vi "Test_Dig_Wfm.vi"(8 "Plot Colors":u32[](array[numeric]), 9 "Threshold Value of a circuit":dbl=30.0, 11 "DataLog":path=path "/Macintosh HD/Users/hasan/My_MAC_Data/3_Dissemination/ICCAD 2016/Experimental_Data/Ckt 8 - Majority Muller C element/kd-0.0135/Majority Muller C_SSADataLog.xls") -> (2 "Close 2":bool)   [LabVIEW 2014]
uses:
  <vilib>/Utility/file.llb/Read From Spreadsheet File (DBL).vi
  <vilib>/Utility/file.llb/Read From Spreadsheet File (string).vi
  <vilib>/Waveform/DTblOps.llb/DTbl Boolean Array to Digital.vi
panel:
  out "size(s)":i32
  out "x/y":dbl
  out "Clr":u32[](array[numeric])
  out "x-scale-multiplier":dbl=10.0
  out "Digital Waveform Graph 2":digitaldata[](graph)
  out "Digital":path
  out "Time":dbl[](array[numeric])
  out "Thres vals":dbl[](array[numeric])
  out "Int Time":i32[](array[numeric])
  out "Idx":i32[](array[numeric])
  out "Q":i32
  out "floor(x/y)":dbl
  out "Plot Names":string[](array[string])=["A", "B", "C", "P0", "P1", "P10", "P11", "P12", "P13", "P2", "P3", "P4", "P5", "P6", "P7", "P8", "P9", "S1", "S2", "S3", "S4", "X", "Y", "Z"]
  out "Mixed Signal Graph":T1(graph)
  out "x > y?":bool[][](array[boolean])
  out "Sp Data":dbl[][](array[numeric]) format="%0.3f"
  in  "Cancel Button":bool
  in  "Close":bool
  in  "Reset":bool
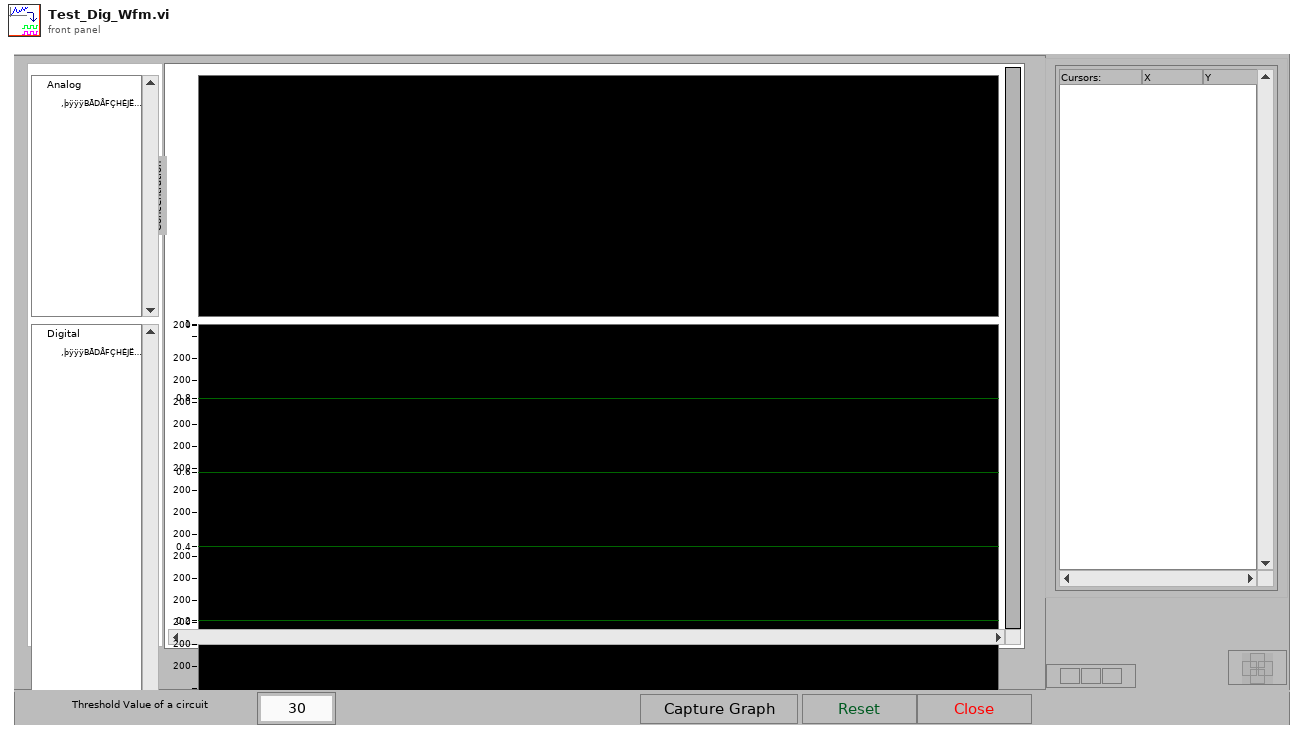
[diagram p1: front panel]
types:
  T1 = cluster{cluster{"Time":i32[], dbl[]}[], digitaldata[]}
  T2 = cluster{cluster{"Int Time":i32[], dbl[]}[], digitaldata[]}
  T3 = cluster{"Color":u32, "PointStyle":u8, "LineStyle":u8, "Interp":u8, "LineWidth":u8, "BarPlotStyle":u8, "FillTo":i16, "XScaleIdx":u32, "YScaleIdx":u32, "Anti-Aliased":bool, "LabelFormat":u8, "TransitionType":u8, "TransitionLocation":u8, "DigitalLineStyle":u8}
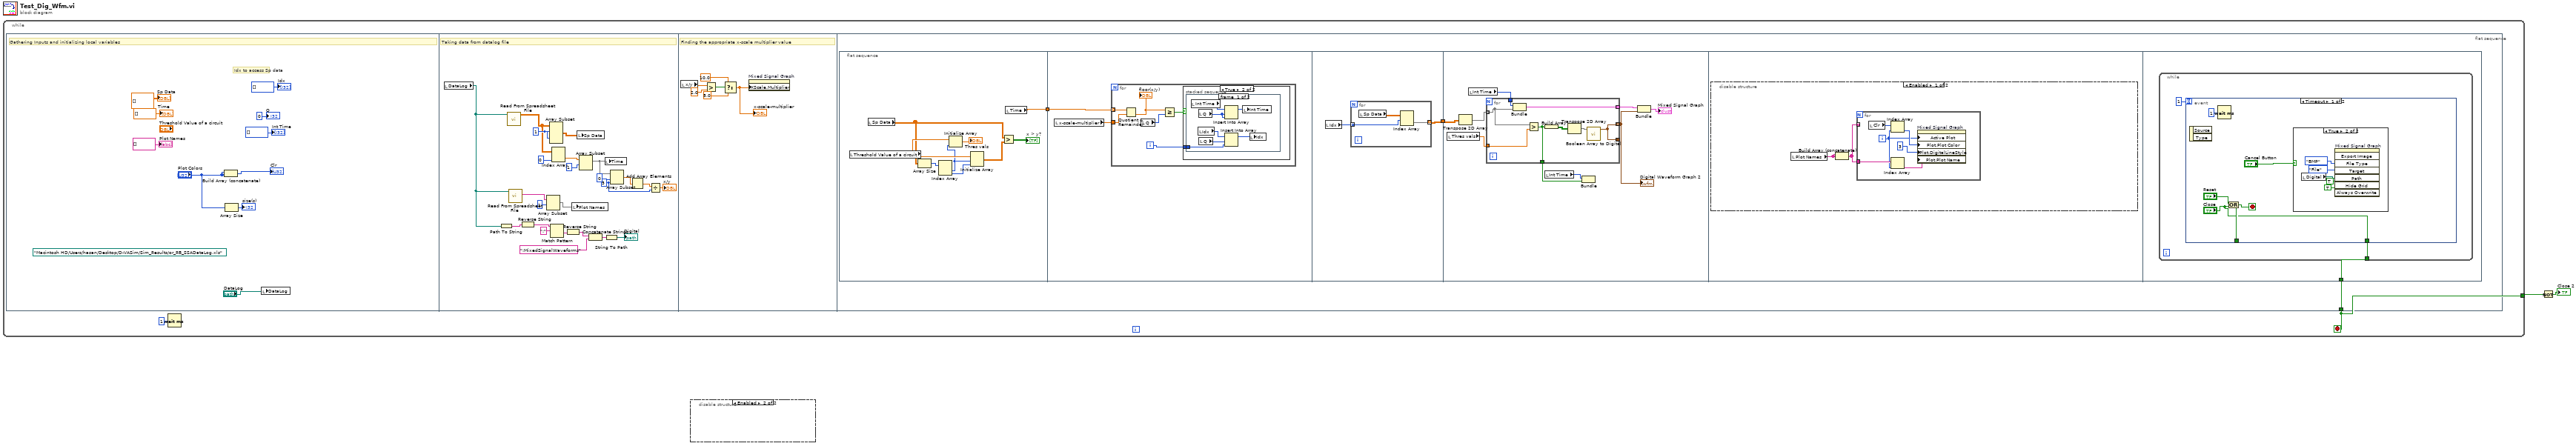
[diagram p0: block diagram]
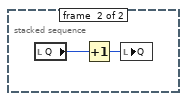
[diagram p3: hidden frame]
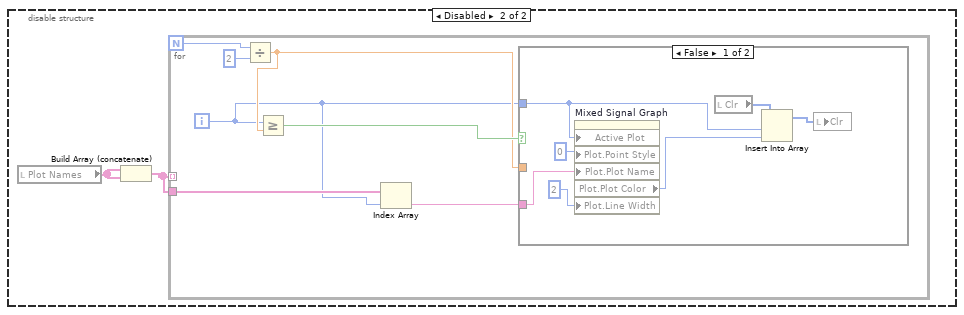
[diagram p4: hidden frame]
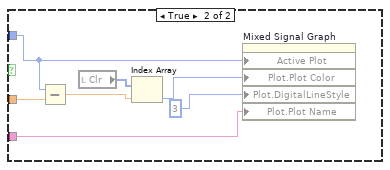
[diagram p5: hidden frame]
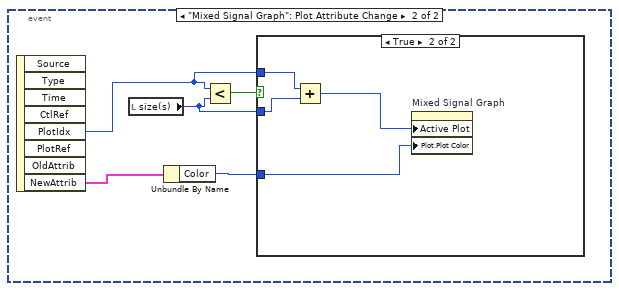
[diagram p7: hidden frame]
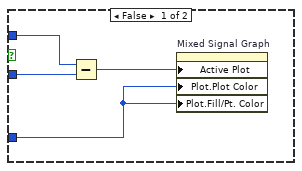
[diagram p8: hidden frame]
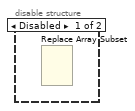
[diagram p9: hidden frame]
diagram:
  n1 = while {
    tunnel: [w3] -> w2
    stop <- w3 stop-if-true
    n2 = flat-sequence {
      tunnel: [w45] -> w3
      frame #0 {
        (unwired) path "/Macintosh HD/Users/hasan/Desktop/D-VASim/Sim_Results/or_RB_SSADataLog.xls" ("DataLog")
        # "Idx to access Sp data"
        # "Gathering Inputs and initializing local variables"
        n3 = Build Array (concatenate)("Plot Colors", "Plot Colors") -> (→"Clr":u32[])
        n4 = Array Size(array="Plot Colors") -> (size(s)=→"size(s)":i32)
        n5 = local write "DataLog"("DataLog") -> ()
        "Sp Data" <- dbl[][] [] ("Sp Data")
        "Plot Names" <- string[] [] ("Plot Names")
        "Time" <- dbl[] [] ("Time")
        "Idx" <- i32[] []
        "Q" <- 0
        "Int Time" <- i32[] []
      }
      frame #1 {
        w16 = 5 ("length")
        w38 = 1 ("index")
        # "Taking data from datalog file"
        n6 = local read "DataLog"() -> (w21:path)
        n7 = Path To String(path=w21) -> (string=w23:string)
        n8 = call-poly <vilib>:"Read From Spreadsheet File.vi"("file path (dialog if empty)"=w21) -> ("all rows"=w36:dbl[][])  [unwired: 6 in, 4 out]
        n9 = call-poly <vilib>:"Read From Spreadsheet File.vi"("file path (dialog if empty)"=w21) -> ("first row"=w32:string[])  [unwired: 6 in, 4 out]
        n10 = Reverse String(1:w23) -> (0:w24:string)
        n11 = Array Subset(array=w32, index=1) -> (w31:string[])  [unwired: 1 in]
        n12 = Array Subset(array=w36, index (row)=w38, index (col)=w38) -> (w37:dbl[][])  [unwired: 2 in]
        n13 = Match Pattern(string=w24, regular expression=":") -> (after substring=w26:string)  [unwired: 1 in, 3 out]
        n14 = Index Array(array=w36, index (col)=0 ("index")) -> (element=w34:dbl[])  [unwired: 1 in]
        n15 = Reverse String(1:w26) -> (0:w27:string)
        n16 = local write "Plot Names"(w31) -> ()
        n17 = local write "Sp Data"(w37) -> ()
        n18 = Array Subset(array=w34, index=1) -> (w20:dbl[])  [unwired: 1 in]
        n19 = Concatenate Strings(w27, ":MixedSignalWaveforms" ("regular expression")) -> (w29:string)
        n20 = local write "Time"(w20) -> ()
        n21 = String To Path(string=w29) -> (path=→"Digital":path)
        n22 = Array Subset(array=w20, index=0, length=w16) -> (w18:dbl[])
        n23 = Add Array Elements(numeric array=w18) -> (sum=w17:dbl)
        n24 = Divide(x=w17, y=w16) -> (x/y=→"x/y":dbl)
      }
      frame #2 {
        # "Finding the appropriate x-scale multiplier value"
        n25 = local read "x/y"() -> (w44:dbl)
        n26 = Greater?(x=w44, y=2.0) -> (0:w42:bool)
        n27 = Select(t=10.0, s=w42, f=5.0) -> (s? t:f=w39:dbl)
        "x-scale-multiplier" <- w39
        n28 = property on="Mixed Signal Graph" class="MixedGraph (strict)"("XScale.Multiplier"=w39) -> ()  [unwired: 2 in, 2 out]
      }
      frame #3 {
        n29 = flat-sequence {
          tunnel: [w56] -> w46
          tunnel: w46 -> [w58]
          tunnel: [w75] -> w47
          tunnel: w47 -> [w85]
          tunnel: [w128] -> w45
          frame #0 {
            n30 = local read "Threshold Value of a circuit"() -> (w55:dbl)
            n31 = local read "Sp Data"() -> (w54:dbl[][])
            n32 = Array Size(array=w54) -> (size(s)=w49:i32[])
            n33 = Index Array(array=w49) -> (element #1=w52:i32, element #2=w48:i32)  [unwired: 2 in]
            n34 = Initialize Array(w55, w52) -> (→"Thres vals":dbl[])
            n35 = Initialize Array(w55, w52, w48) -> (w50:dbl[][])
            n36 = Greater?(x=w54, y=w50) -> (0:→"x > y?":bool[][])
            n37 = local read "Time"() -> (w56:dbl[])
          }
          frame #1 {
            n38 = local read "x-scale-multiplier"() -> (w57:dbl)
            n39 = for {
              tunnel: w58 -> [w64] mode=indexing
              tunnel: w57 -> [w61]
              i -> [w62]
              n40 = Quotient & Remainder(x=w64, y=w61) -> (floor(x/y)=w60:dbl)  [unwired: 1 out]
              "floor(x/y)" <- w60
              n41 = local read "Q"() -> (w59:i32)
              n42 = Greater Or Equal?(x=w60, y=w59) -> (x >= y?=w63:bool)
              n43 = case shown="True" w63 {
                tunnel: w62 -> [_ w65]
                frame False {
                }
                frame True {
                  n44 = stacked-sequence {
                    tunnel: w65 -> [w66 _]
                    frame #0 {
                      n45 = local read "Int Time"() -> (w72:i32[])
                      n46 = local read "Idx"() -> (w67:i32[])
                      n47 = local read "Q"() -> (w70:i32)
                      n48 = local read "Q"() -> (w69:i32)
                      n49 = Insert Into Array(array=w72, index=w70, new element=w70) -> (w71:i32[])
                      n50 = Insert Into Array(array=w67, index=w69, new element=w66) -> (w68:i32[])
                      n51 = local write "Int Time"(w71) -> ()
                      n52 = local write "Idx"(w68) -> ()
                    }
                    frame #1 {
                      n53 = local read "Q"() -> (w74:i32)
                      n54 = Increment(x=w74) -> (x+1=w73:i32)
                      n55 = local write "Q"(w73) -> ()
                    }
                  }
                }
              }
            }
          }
          frame #2 {
            n56 = local read "Idx"() -> (w76:i32[])
            n57 = for {
              tunnel: w76 -> [w78] mode=indexing
              tunnel: [w77] -> w75 mode=indexing
              n58 = local read "Sp Data"() -> (w79:dbl[][])
              n59 = Index Array(array=w79, index (row)=w78) -> (element=w77:dbl[])  [unwired: 1 in]
            }
          }
          frame #3 {
            n60 = local read "Thres vals"() -> (w88:dbl[])
            n61 = Transpose 2D Array(2D array=w85) -> (transposed array=w87:dbl[][])
            n62 = local read "Int Time"() -> (w84:i32[])
            n63 = for {
              tunnel: w87 -> [w92] mode=indexing
              tunnel: [w96] -> w86 mode=indexing
              tunnel: w88 -> [w95]
              tunnel: [w90] -> w80 mode=indexing
              tunnel: w84 -> [w91]
              tunnel: [w90] -> _
              tunnel: [w89] -> w81
              n64 = Bundle("Int Time"=w91, w92) -> (w96:cluster{"Int Time":i32[], dbl[]})  [unwired: 1 in]
              n65 = Greater?(x=w92, y=w95) -> (0:w89:bool[])
              n66 = Build Array(w89) -> (w94:bool[][])
              n67 = Transpose 2D Array(2D array=w94) -> (transposed array=w93:bool[][])
              n68 = call-poly <vilib>:"Boolean Array to Digital.vi"("boolean array"=w93) -> ("digital data"=w90:digitaldata)  [unwired: 9 in, 1 out]
            }
            "Digital Waveform Graph 2" <- w80
            n69 = local read "Int Time"() -> (w82:i32[])
            n70 = Bundle("Int Time"=w82, w81) -> ()  [unwired: 1 in, 1 out]
            n71 = Bundle(w86, w80) -> (→"Mixed Signal Graph":T2)  [unwired: 1 in]
          }
          frame #4 {
            n72 = disable-structure shown="Enabled" {
              frame Enabled {
                n73 = local read "Plot Names"() -> (w98:string[])
                n74 = Build Array (concatenate)(w98, w98) -> (w97:string[])
                n75 = for {
                  tunnel: w97 -> [_] mode=indexing
                  tunnel: w97 -> [w101]
                  i -> [w100]
                  n76 = local read "Clr"() -> (w104:u32[])
                  n77 = Index Array(array=w104, index=w100) -> (element=w103:u32)
                  n78 = Index Array(array=w101, index=w100) -> (element=w99:string)
                  n79 = property on="Mixed Signal Graph" class="MixedGraph (strict)"("Active Plot"=w100, "Plot.Plot Color"=w103, "Plot.DigitalLineStyle"=u8 3 ("Plot.Line Style"), "Plot.Plot Name"=w99) -> ()  [unwired: 2 in, 2 out]
                }
              }
              frame Disabled {
                n80 = local read "Plot Names"() -> (w106:string[])
                n81 = Build Array (concatenate)(w106, w106) -> (w105:string[])
                n82 = for {
                  N -> [w113]
                  tunnel: w105 -> [_] mode=indexing
                  tunnel: w105 -> [w109]
                  i -> [w108]
                  n83 = Divide(x=w113, y=2) -> (x/y=w110:dbl)
                  n84 = Greater Or Equal?(x=w108, y=w110) -> (x >= y?=w111:bool)
                  n85 = Index Array(array=w109, index=w108) -> (element=w107:string)
                  n86 = case shown="False" w111 {
                    tunnel: w108 -> [w118 w126]
                    tunnel: w110 -> [_ w125]
                    tunnel: w107 -> [w115 w121]
                    frame False {
                      n87 = property on="Mixed Signal Graph" class="MixedGraph (strict)"("Active Plot"=w118, "Plot.Point Style"=u8 0, "Plot.Plot Name"=w115, "Plot.Line Width"=u8 2) -> ("Plot.Plot Color"=w116:u32)  [unwired: 2 in, 2 out]
                      n88 = local read "Clr"() -> (w119:u32[])
                      n89 = Insert Into Array(array=w119, index=w118, new element=w116) -> (w120:u32[])
                      n90 = local write "Clr"(w120) -> ()
                    }
                    frame True {
                      n91 = Subtract(x=w126, y=w125) -> (x-y=w124:dbl)
                      n92 = local read "Clr"() -> (w127:u32[])
                      n93 = Index Array(array=w127, index=w124) -> (element=w123:u32)
                      n94 = property on="Mixed Signal Graph" class="MixedGraph (strict)"("Active Plot"=w126, "Plot.Plot Color"=w123, "Plot.DigitalLineStyle"=u8 3 ("Plot.Line Style"), "Plot.Plot Name"=w121) -> ()  [unwired: 2 in, 2 out]
                    }
                  }
                }
              }
            }
          }
          frame #5 {
            n95 = while {
              tunnel: [w130] -> w128
              stop <- w131 stop-if-true
              n96 = event shown="[0] Timeout" {
                selector: _ -> [_ _]
                dyn-events: _ -> [_ _]
                timeout: 1 -> [_ _]
                tunnel: [w135 _] -> w131
                tunnel: ["Close" _] -> w130
                event Timeout {
                  n97 = event-data() -> ()  [unwired: 1 in, 2 out]
                  n98 = Wait (ms)(milliseconds to wait=u32 1) -> ()  [unwired: 1 out]
                  n99 = Or(x="Reset", y="Close") -> (x .or. y?=w135:bool)
                  n100 = case shown="True" "Cancel Button" {
                    frame False {
                    }
                    frame True {
                      n101 = local read "Digital"() -> (w141:path)
                      n102 = invoke on="Mixed Signal Graph" class="MixedGraph (strict)" method="Export Image"("File Type"=enum32{"BMP", "EPS", "EMF", "PICT"}."BMP", "Target"=enum32{"File", "Clipboard"}."File", "Path"=w141, "Hide Grid"=TRUE, "Always Overwrite"=TRUE) -> ()  [unwired: 3 in, 8 out]
                    }
                  }
                }
                event "Mixed Signal Graph": Plot Attribute Change {
                  n103 = event-data() -> ("PlotIdx"=w144:i32, "NewAttrib"=w143:T3)  [unwired: 1 in, 6 out]
                  n104 = local read "size(s)"() -> (w145:i32)
                  n105 = Unbundle By Name(w143) -> ("Color"=w142:u32)
                  n106 = Less?(x=w144, y=w145) -> (x < y?=w146:bool)
                  n107 = case shown="True" w146 {
                    tunnel: w145 -> [w149 w154]
                    tunnel: w144 -> [w148 w153]
                    tunnel: w142 -> [w147 w151]
                    frame False {
                      n108 = Subtract(x=w148, y=w149) -> (x-y=w150:i32)
                      n109 = property on="Mixed Signal Graph" class="MixedGraph (strict)"("Active Plot"=w150, "Plot.Plot Color"=w147, "Plot.Fill/Pt. Color"=w147) -> ()  [unwired: 2 in, 2 out]
                    }
                    frame True {
                      n110 = Add(x=w153, y=w154) -> (x+y=w152:i32)
                      n111 = property on="Mixed Signal Graph" class="MixedGraph (strict)"("Active Plot"=w152, "Plot.Plot Color"=w151) -> ()  [unwired: 2 in, 2 out]
                    }
                  }
                }
              }
            }
          }
        }
      }
    }
    n112 = Wait (ms)(milliseconds to wait=u32 1) -> ()  [unwired: 1 out]
  }
  n113 = disable-structure shown="Enabled" {
    frame Disabled {
      n114 = Replace Array Subset() -> ()  [unwired: 4 in, 1 out]
    }
    frame Enabled {
    }
  }
  n115 = Not(x=w2) -> (.not. x?=→"Close 2":bool)
